vi "PIC_RFFE_Initialize Updated.vi"(8 "error in":errorcluster, 11 "VISA In":refnum<visa-resource-name>) -> (0 "error out":errorcluster, 3 "VISA Out":refnum<visa-resource-name>)   [LabVIEW 2017]
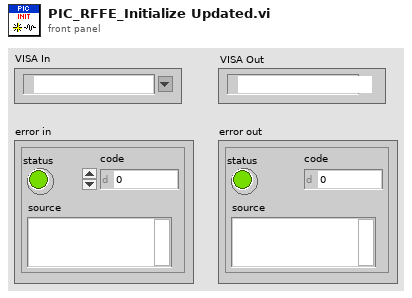
[diagram p1: front panel]
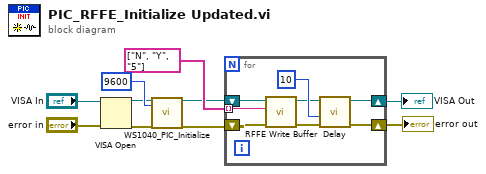
[diagram p0: block diagram]
diagram:
  n1 = VISA Open(error in (no error)="error in", VISA resource name="VISA In") -> (VISA resource name=w2:refnum<visa-resource-name>, error out=w3:errorcluster)  [unwired: 3 in]
  n2 = call "WS1040_PIC_Initialize.vi"("COM_In"=w2, "baud rate (9600)"=u32 9600, "error in (no error)"=w3) -> ("COM_Out"=w1:refnum<visa-resource-name>, "error out"=w4:errorcluster)  [unwired: 15 in]
  n3 = for {
    tunnel: string[] ["N", "Y", "5"] -> [w13] mode=indexing
    shift-right: [w17] -> w8
    shift-left: w4 -> [w12]
    shift-right: [w11] -> w9
    shift-left: w1 -> [w14]
    n4 = call "RFFE Write Buffer.vi"("error in (no error)"=w12, "write buffer"=w13, "VISA resource name"=w14) -> ("error out"=w15:errorcluster, "VISA resource name out"=w11:refnum<visa-resource-name>)  [unwired: 7 in]
    n5 = call "Delay.vi"("error in (no error)"=w15, "Delay"=u32 10) -> ("error out"=w17:errorcluster)  [unwired: 9 in]
  }
  "VISA Out" <- w9
  "error out" <- w8
